vi "ArmBegin2.vi"   [LabVIEW 2023]
doc: "Arm begin\nOpens ArmLift motor\nInputs:\nNone\nOutputs:\nnone"
uses:
  <vilib>/Rock Robotics/WPI/ThirdParty/REV Robotics/REVLib/Typedef/Spark MAX Motor Type.ctl
  <vilib>/Rock Robotics/WPI/ThirdParty/REV Robotics/REVLib/Typedef/Spark MAX Idle Mode.ctl
types:
  T1 = typedef "Spark MAX Idle Mode.ctl" = enum16{"Coast", "Brake"}
  T2 = typedef "Spark MAX Motor Type.ctl" = enum16{"Brushed", "Brushless"}
  T3 = typedef "WPI_MotorControlDeviceRef.ctl" = cluster{"DeviceStatus":errorcluster, "Type":T4, "PWM":cluster{"PWM Channel":T5, "DeadBand":T6}, "CAN":cluster{"Device Number":u8, "SetOutput VI Ref":variant, "GetOutput VI Ref":variant, "Enable VI Ref":variant, "Disable VI Ref":variant, "Data":variant}, "Invert":bool, "DIO PWM":cluster{"PWM \"Enable\" Channel":T5, "DIOChannel":T7, "PWM Rate":dbl}}
  T4 = typedef "WPI_MotorControlType.ctl" = enum16{"PWM", "CAN", "DIO PWM"}
  T5 = typedef "FPGA_DIOPWMChannel.ctl" = enum8{"PWM 0", "PWM 1", "PWM 2", "PWM 3", "PWM 4", "PWM 5", "PWM 6", "PWM 7", "PWM 8", "PWM 9", "PWM MXP 0", "PWM MXP 1", "PWM MXP 2", "PWM MXP 3", "PWM MXP 4", "PWM MXP 5", "PWM MXP 6", "PWM MXP 7", "PWM MXP 8", "PWM MXP 9", "Invalid"}
  T6 = typedef "WPI_PWMDeadband.ctl" = cluster{"Name":string, "maxPositivePwm":i32, "minPositivePwm":i32, "centerPwm":i32, "maxNegativePwm":i32, "minNegativePwm":i32, "angularRange":u16}
  T7 = typedef "FPGA_DIOChannel.ctl" = enum8{"DIO 0", "DIO 1", "DIO 2", "DIO 3", "DIO 4", "DIO 5", "DIO 6", "DIO 7", "DIO 8", "DIO 9", "DIO MXP 0", "DIO MXP 1", "DIO MXP 2", "DIO MXP 3", "DIO MXP 4", "DIO MXP 5", "DIO MXP 6", "DIO MXP 7", "DIO MXP 8", "DIO MXP 9", "DIO MXP 10", "DIO MXP 11", "DIO MXP 12", "DIO MXP 13", "DIO MXP 14", "DIO MXP 15", "SPI Port CS1", "SPI Port CS2", "SPI Port CS3", "SPI Port MISO", "SPI Port MOSI", "Invalid"}
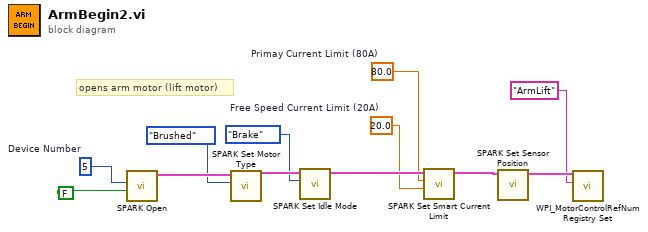
[diagram p0: block diagram]
diagram:
  w4 = 20.0  # Free Speed Current Limit (20A)
  w5 = 80.0  # Primay Current Limit (80A)
  w12 = u8 5  # Device Number
  # "opens arm motor (lift motor)"
  n1 = call <vilib>:"SPARK Open.vi"("Invert"=FALSE, "Device Number"=w12) -> ("MotorControlDeviceRef"=w10:T3)  [unwired: 8 in, 1 out]
  n2 = call <vilib>:"SPARK Set Motor Type.vi"("Motor Type"=Spark_MAX_Motor_Type."Brushed", "MotorControlDevRef"=w10) -> ("MotorControlDeviceRef"=w8:T3)  [unwired: 8 in, 1 out]
  n3 = call <vilib>:"SPARK Set Idle Mode.vi"("Idle Mode"=Spark_MAX_Idle_Mode."Brake", "MotorControlDeviceRef in"=w8) -> ("MotorControlDeviceRef out"=w6:T3)  [unwired: 8 in, 1 out]
  n4 = call <vilib>:"SPARK Set Smart Current Limit.vi"("Free Speed Current Limit (20A)"=w4, "Primay Current Limit (80A)"=w5, "MotorControlDeviceRef in"=w6) -> ("MotorControlDeviceRef out"=w3:T3)  [unwired: 7 in, 1 out]
  n5 = call <vilib>:"SPARK Set Sensor Position.vi"("MotorControlDeviceRef"=w3) -> ("MotorControlDeviceRef"=w2:T3)  [unwired: 9 in, 1 out]
  n6 = call <vilib>:"WPI_MotorControlRefNum Registry Set.vi"("refnum name"="ArmLift", "MotorControlDevRef"=w2) -> ()  [unwired: 8 in, 2 out]
